vi "aquire_FPS.vi"(7 "Time Value In /ms":u32) -> (8 "Time Value Out /ms":u32, 12 "Execution time / ms":u32, 14 "FPS":dbl)   [LabVIEW 2023]
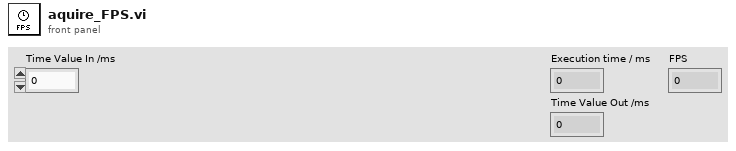
[diagram p1: front panel]
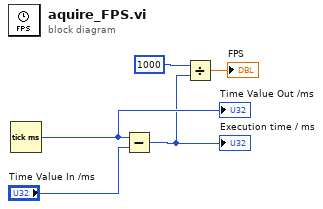
[diagram p0: block diagram]
diagram:
  n1 = Tick Count (ms)() -> (millisecond timer value=w5:u32)
  "Time Value Out /ms" <- w5
  n2 = Subtract(x=w5, y="Time Value In /ms") -> (x-y=w1:u32)
  "Execution time / ms" <- w1
  n3 = Divide(x=u32 1000 ("y"), y=w1) -> (x/y=→"FPS":dbl)
